vi "ping.vi"(8 "error in":errorcluster, 9 "timeout":dbl=1000.0, 10 "count":dbl=1.0, 11 "host":string="localhost") -> (0 "error out":errorcluster, 3 "found":bool)   [LabVIEW 2014]
panel:
  out "standard output":string
  out "IP":string
  out "return code":i32
  out "resulting string":string
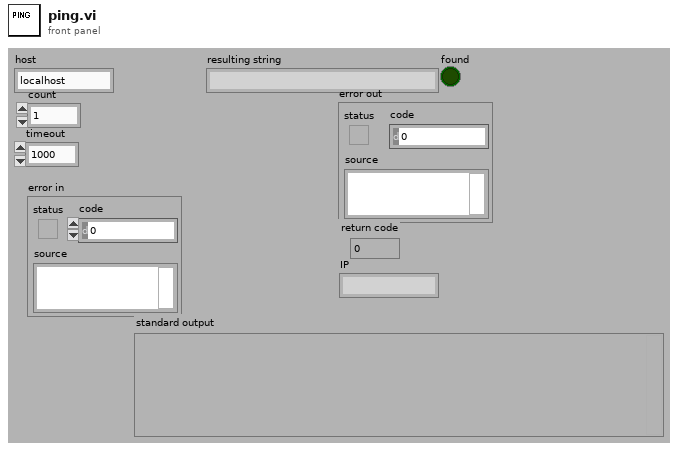
[diagram p1: front panel]
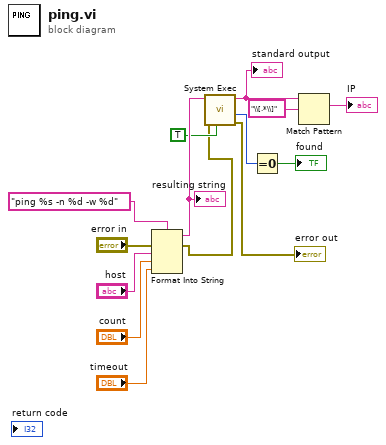
[diagram p0: block diagram]
diagram:
  n1 = Format Into String(format string="ping %s -n %d -w %d", error in="error in", "host", "count", "timeout") -> (resulting string=w7:string, error out=w2:errorcluster)  [unwired: 1 in]
  "resulting string" <- w7
  n2 = call <vilib>:"System Exec.vi"("run minimized? (F)"=TRUE, "error in (no error)"=w2, "command line"=w7) -> ("error out"=→"error out":errorcluster, "return code"=w9:i32, "standard output"=w6:string)  [unwired: 3 in, 3 out]
  "standard output" <- w6
  n3 = Equal To 0?(x=w9) -> (x = 0?=→"found":bool)
  n4 = Match Pattern(string=w6, regular expression="\\[.*\\]") -> (match substring=→"IP":string)  [unwired: 4 out]
